vi "Read Async Elements.vi"(10 "Async Elements":refnum<class "Async Elements.lvclass">) -> (2 "Async Elements":refnum<queue>)   [LabVIEW 2025, in "jettl.lvlib" / "Base Async Elements.lvlib"]
uses:
  Base Async Elements.lvlib
  Async Elements.ctl
  Async Elements/Async Elements.lvclass
  Base Async Elements/Base Async Elements.lvclass
  Attributes/Attributes.lvclass
  jettl.lvlib
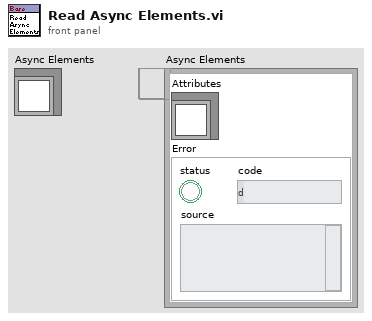
[diagram p1: front panel]
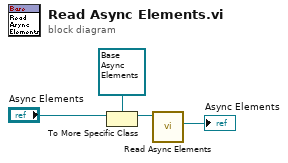
[diagram p0: block diagram]
diagram:
  n1 = To More Specific Class(target class=refnum<class "Base Async Elements.lvclass"> refnum ("jettl.lvlib:Base Async Elements.lvlib:Base Async Elements.lvclass"), reference="Async Elements") -> (specific class reference=w3:refnum<class "Base Async Elements.lvclass">)  [unwired: 1 in, 1 out]
  n2 = call "Read Async Elements.vi"("Base Async Elements in"=w3) -> ("Async Elements"=→"Async Elements":refnum<queue>)  [unwired: 10 in]
